vi "JsonFile_GetAttribute(String).vi"(8 "error in (no error)":errorcluster, 9 "Default Value":string, 10 "Attribute":string, 11 "Json":path) -> (0 "error out":errorcluster, 1 "Found?":bool, 2 "Value":string, 3 "Json":path)   [LabVIEW 2019, in "lv-apt-json-file.lvlib"]
uses:
  <userlib>/_lvAPT/lv-apt-json-file/lv-apt-json-file.lvlib
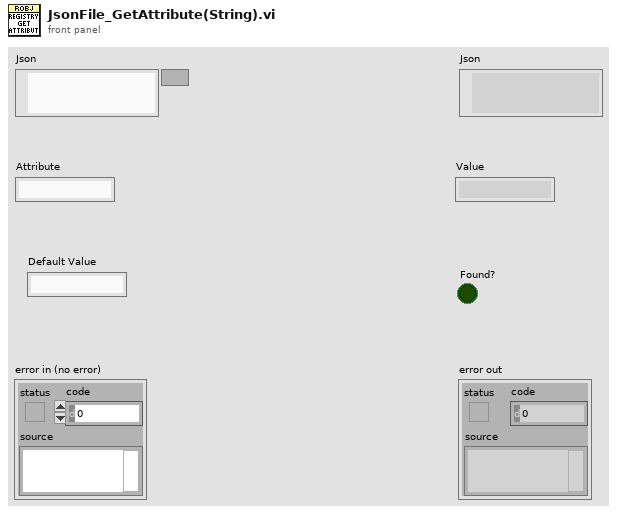
[diagram p1: front panel]
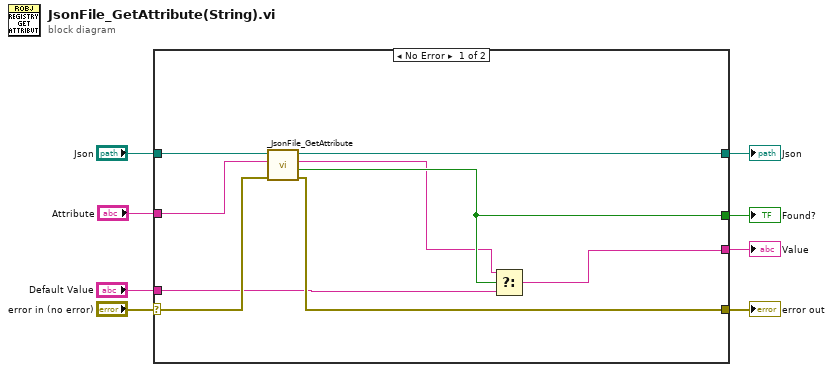
[diagram p0: block diagram]
diagram:
  n1 = case shown="No Error" "error in (no error)" {
    selector: "error in (no error)" -> [w15 w19]
    tunnel: "Json" -> [w16 w18]
    tunnel: "Attribute" -> [w17 _]
    tunnel: [w14 w18] -> w6
    tunnel: [w13 w19] -> w4
    tunnel: [w12 _] -> w3
    tunnel: [w10 _] -> w2
    tunnel: "Default Value" -> [w11 _]
    frame No Error {
      n2 = call <userlib>:"_JsonFile_GetAttribute.vi"("error in (no error)"=w15, "Attribute"=w17, "Json"=w16) -> ("error out"=w13:errorcluster, "Found?"=w12:bool, "String"=w9:string, "Json (dup)"=w14:path)  [unwired: 5 in]
      n3 = Select(t=w9, s=w12, f=w11) -> (s? t:f=w10:string)
    }
    frame Error {
    }
  }
  "error out" <- w4
  "Json" <- w6
  "Value" <- w2
  "Found?" <- w3
